vi "init.vi"(8 "error in (no error)":errorcluster, 11 "NYStyleCheesePizza in":refnum<class "ChicagoStylePepperoniPizza.lvclass">) -> (0 "error out":errorcluster, 3 "NYStyleCheesePizza out":refnum<class "ChicagoStylePepperoniPizza.lvclass">)   [LabVIEW 2021, in "ChicagoStylePepperoniPizza.lvclass"]
uses:
  ChicagoStylePepperoniPizza.lvclass
  ChicagoStylePepperoniPizza.lvclass/ChicagoStylePepperoniPizza.ctl
panel:
  # "Connector Pane"
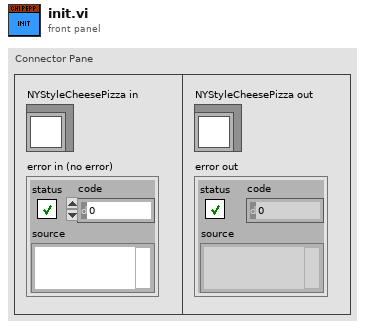
[diagram p1: front panel]
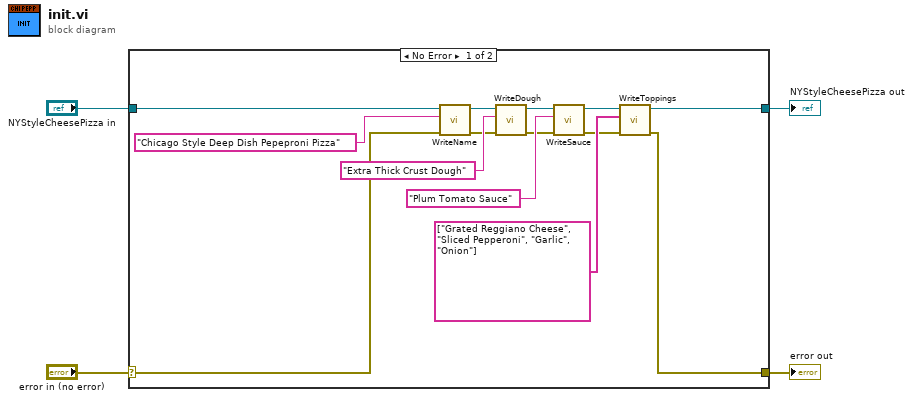
[diagram p0: block diagram]
diagram:
  n1 = case shown="No Error" "error in (no error)" {
    selector: "error in (no error)" -> [w6 w20]
    tunnel: [w5 w20] -> w3
    tunnel: [w11 w19] -> w1
    tunnel: "NYStyleCheesePizza in" -> [w16 w19]
    frame No Error {
      n2 = call-dynamic "WriteName.vi"("error in (no error)"=w6, "name"="Chicago Style Deep Dish Pepeproni Pizza", "object in"=w16) -> ("error out"=w9:errorcluster, "object out"=w15:refnum<class "ChicagoStylePepperoniPizza.lvclass">)  [unwired: 7 in]
      n3 = call-dynamic "WriteDough.vi"("error in (no error)"=w9, "dough"="Extra Thick Crust Dough", "object in"=w15) -> ("error out"=w8:errorcluster, "object out"=w14:refnum<class "ChicagoStylePepperoniPizza.lvclass">)  [unwired: 7 in]
      n4 = call-dynamic "WriteSauce.vi"("error in (no error)"=w8, "sauce"="Plum Tomato Sauce", "object in"=w14) -> ("error out"=w7:errorcluster, "object out"=w12:refnum<class "ChicagoStylePepperoniPizza.lvclass">)  [unwired: 7 in]
      n5 = call-dynamic "WriteToppings.vi"("error in (no error)"=w7, "toppings"=string[] ["Grated Reggiano Cheese", "Sliced Pepperoni", "Garlic", "Onion"], "object in"=w12) -> ("error out"=w5:errorcluster, "object out"=w11:refnum<class "ChicagoStylePepperoniPizza.lvclass">)  [unwired: 7 in]
    }
    frame Error {
    }
  }
  "error out" <- w3
  "NYStyleCheesePizza out" <- w1
